vi "Autonomous Independent.vi"() -> ()   [LabVIEW 2014]
doc: "This VI is called when autonomous begins, and will automatically be terminated when autonomous ends. You can carry out timed or sensor driven robot movement independently without needing to return to the caller."
uses:
  Robot Global Data.vi
  <vilib>/Rock Robotics/Network Tables/NT Read Numeric Array.vi
  900/SwerveDrive/SwerveDriveRotate.vi
  <vilib>/Rock Robotics/WPI/CAN/TalonSRX/WPI_CANTalonSRX_APIControlMode.ctl
  <vilib>/Rock Robotics/Network Tables/NT Read Boolean Array.vi
  <vilib>/Rock Robotics/Network Tables/NT Read Number.vi
  <vilib>/Rock Robotics/Network Tables/NT Read Boolean.vi
panel:
  in  "Reverse Pivot Limit":dbl=-512.0
  in  "Forward Pivot Limit":dbl
  in  "Target X":dbl=103.5 format="%#_13g"
  # "Be sure to right-click and choose Data Operations>>Make Current Value default if you want to save the array values with the VI"
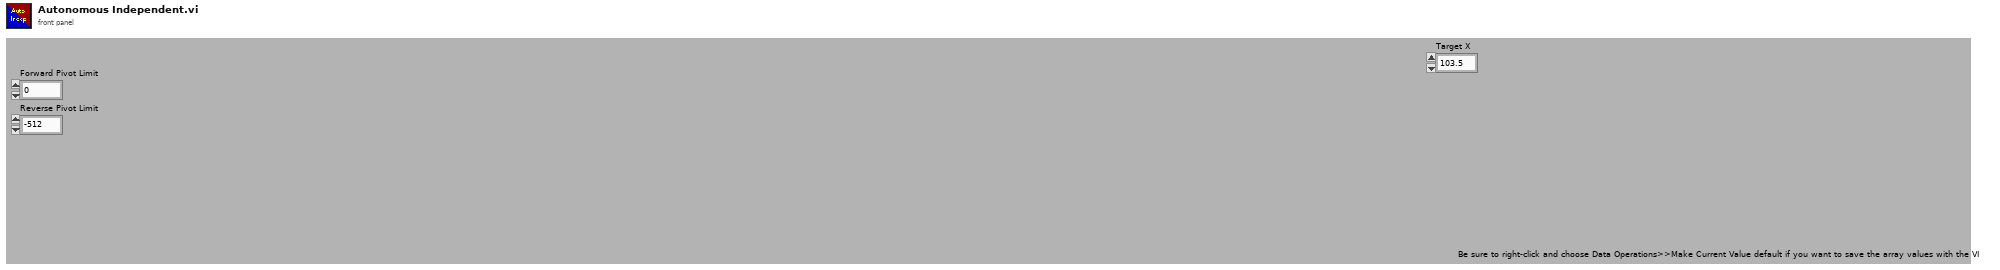
[diagram p1: front panel]
types:
  T1 = enum16{"Open", "Close", "Continue", "Stop", "Toggle"}
  T2 = typedef "WPI_CANTalonSRX_APIControlMode.ctl" = enum8{"Percent VBus", "Speed", "Position", "Slave", "Unchanged / Invalid"}
  T3 = typedef "WPI_MotorControlDeviceRef.ctl" = cluster{"DeviceStatus":errorcluster, "Type":T4, "PWM":cluster{"Controller":T5, "PWM Channel":T6, "DeadBand":T7}, "CAN":cluster{"Device Number":u8, "Control Mode":T8, "Semaphore":T9, "Max Vout":dbl, "TalonSRX Control Mode":T2}, "Invert":bool, "TransformRef":T10, "InvTransformRef":T10}
  T4 = typedef "WPI_MotorControlType.ctl" = enum16{"PWM", "CAN", "CANTalonSRX"}
  T5 = typedef "FPGA_TypedefDigitalModule.ctl" = enum16{"Controller 1"}
  T6 = typedef "FPGA_DIOPWMChannel.ctl" = enum8{"PWM 0", "PWM 1", "PWM 2", "PWM 3", "PWM 4", "PWM 5", "PWM 6", "PWM 7", "PWM 8", "PWM 9", "PWM MXP 0", "PWM MXP 1", "PWM MXP 2", "PWM MXP 3", "PWM MXP 4", "PWM MXP 5", "PWM MXP 6", "PWM MXP 7", "PWM MXP 8", "PWM MXP 9", "Invalid"}
  T7 = typedef "WPI_PWMDeadband.ctl" = cluster{"Name":string, "maxPositivePwm":i32, "minPositivePwm":i32, "centerPwm":i32, "maxNegativePwm":i32, "minNegativePwm":i32, "angularRange":u16}
  T8 = typedef "WPI_CANJaguar_ControlMode.ctl" = enum8{"Percent VBus", "Current", "Speed", "Position", "Voltage"}
  T9 = typedef "Semaphore RefNum" = refnum<k1>
  T10 = typedef "WPI_PWMTransform_ConPane.ctl" = refnum<vi>
  T11 = typedef "WPI_CANTalonSRX_GlobalStatus.ctl" = cluster{"Applied Throttle":dbl, "Module Enabled":bool, "CAN Error":errorcluster, "Closed Loop Error":dbl, "Forward Limit Switch Closed":bool, "Reverse Limit Switch Closed":bool, "Sensor Position":dbl, "Sensor Velocity":dbl, "Current":dbl, "Sticky Fault - Over Temp":bool, "Sticky Fault - Under Voltage":bool, "Sticky Fault - Forward Limit":bool, "Sticky Fault - Reverse Limit":bool, "Sticky Fault - Forward Soft Limit":bool, "Sticky Fault - Reverse Soft Limit":bool, "Brake is Enabled":bool, "Encoder Position":dbl, "Encoder Velocity":dbl, "Encoder Index Count":dbl, "Encoder A Pin State":bool, "Encoder B Pin State":bool, "Encoder Index Pin State":bool, "Analog In":dbl, "Analog In Velocity":dbl, "Temperature (C)":dbl, "Battery Voltage":dbl}
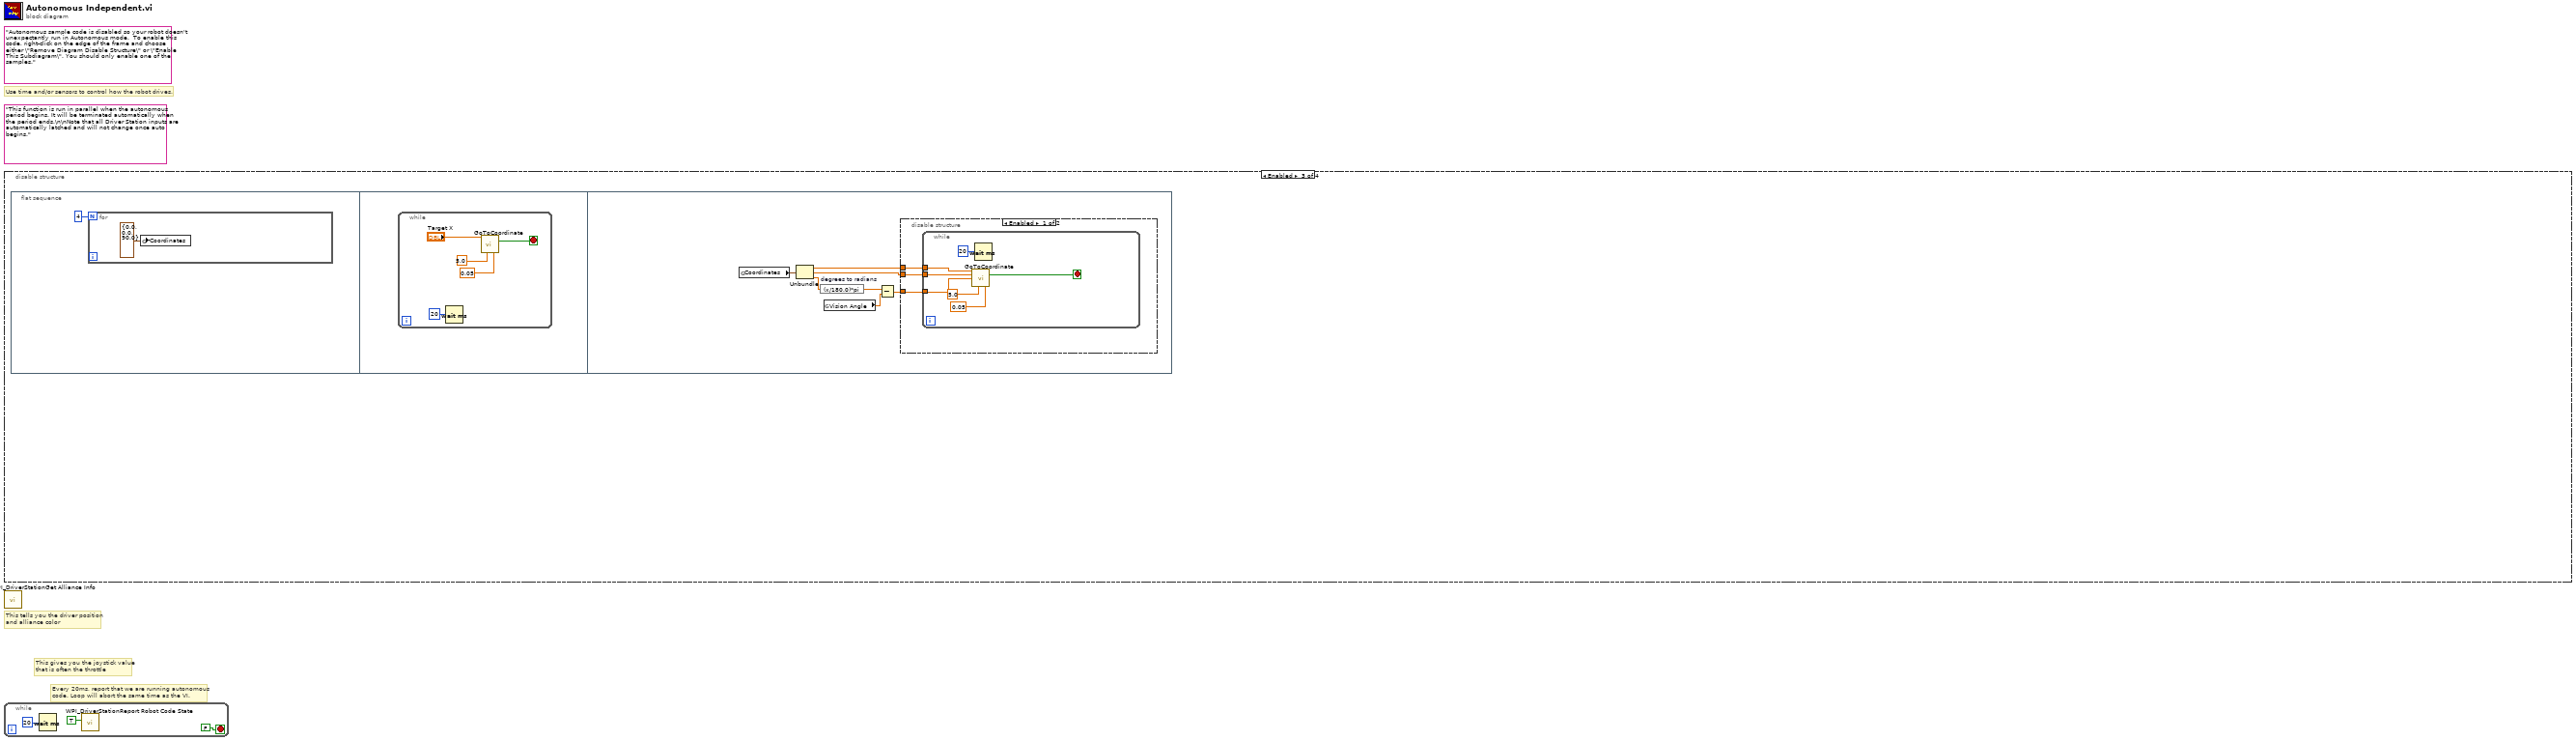
[diagram p0: block diagram]
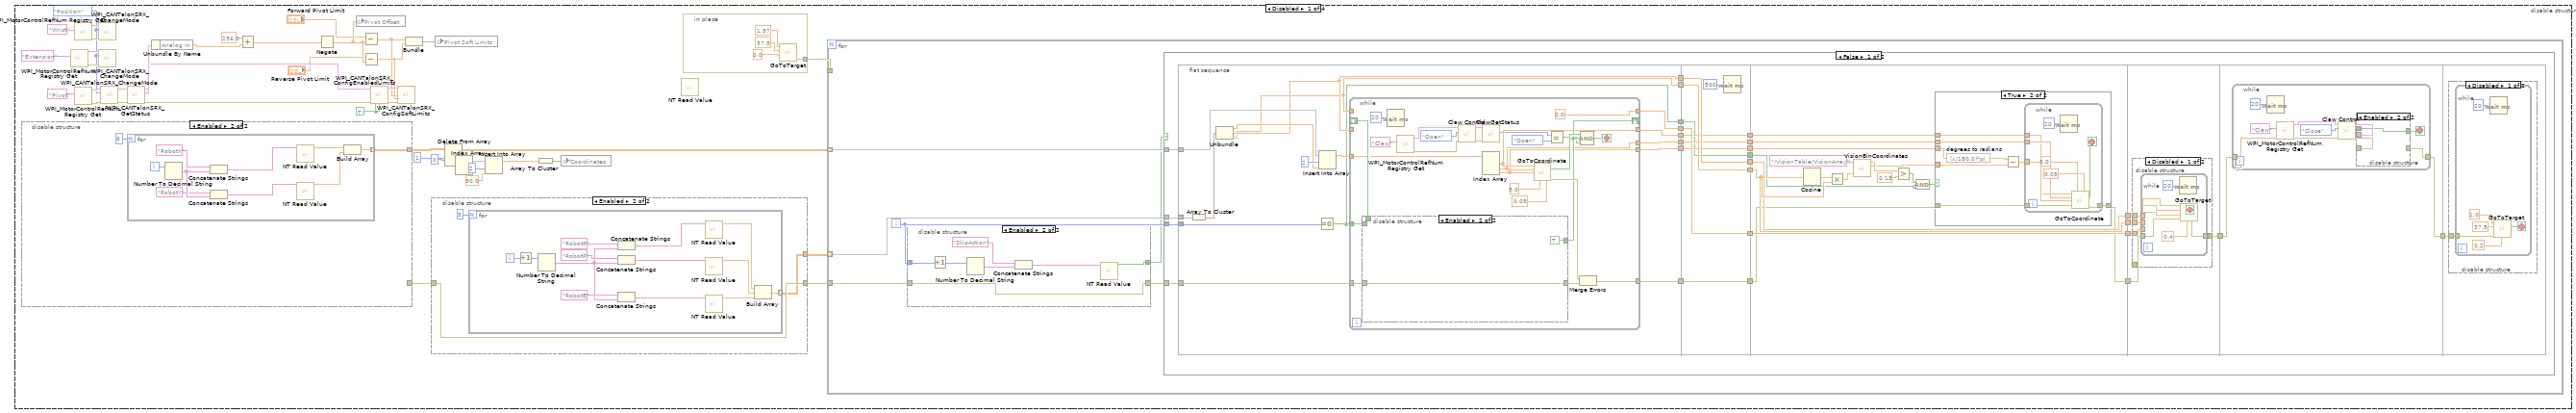
[diagram p2: hidden frame]
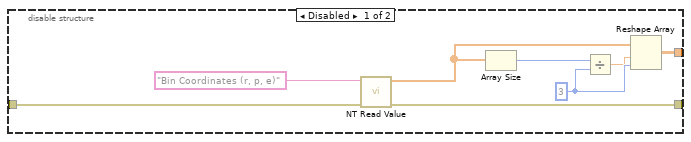
[diagram p3: hidden frame]
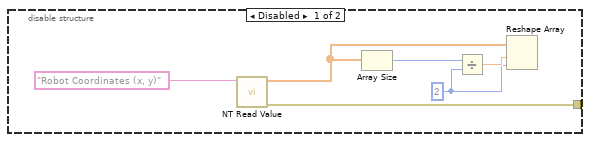
[diagram p4: hidden frame]
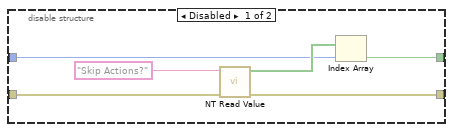
[diagram p5: hidden frame]
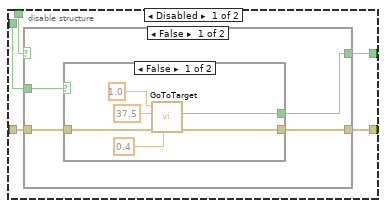
[diagram p6: hidden frame]
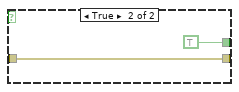
[diagram p7: hidden frame]
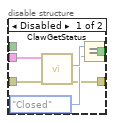
[diagram p11: hidden frame]
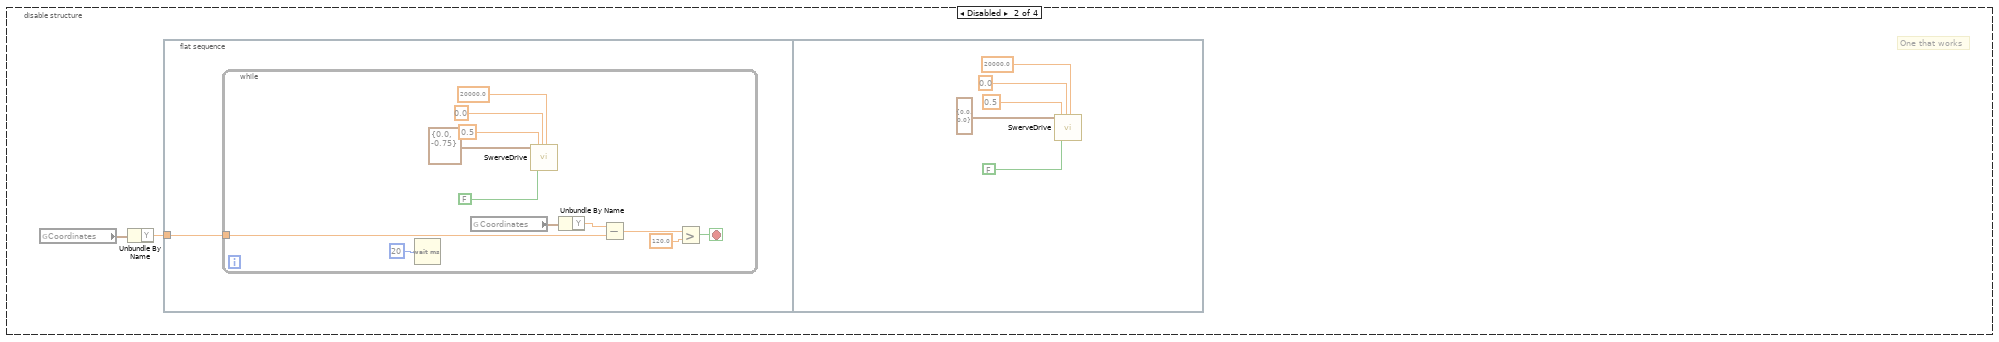
[diagram p14: hidden frame]
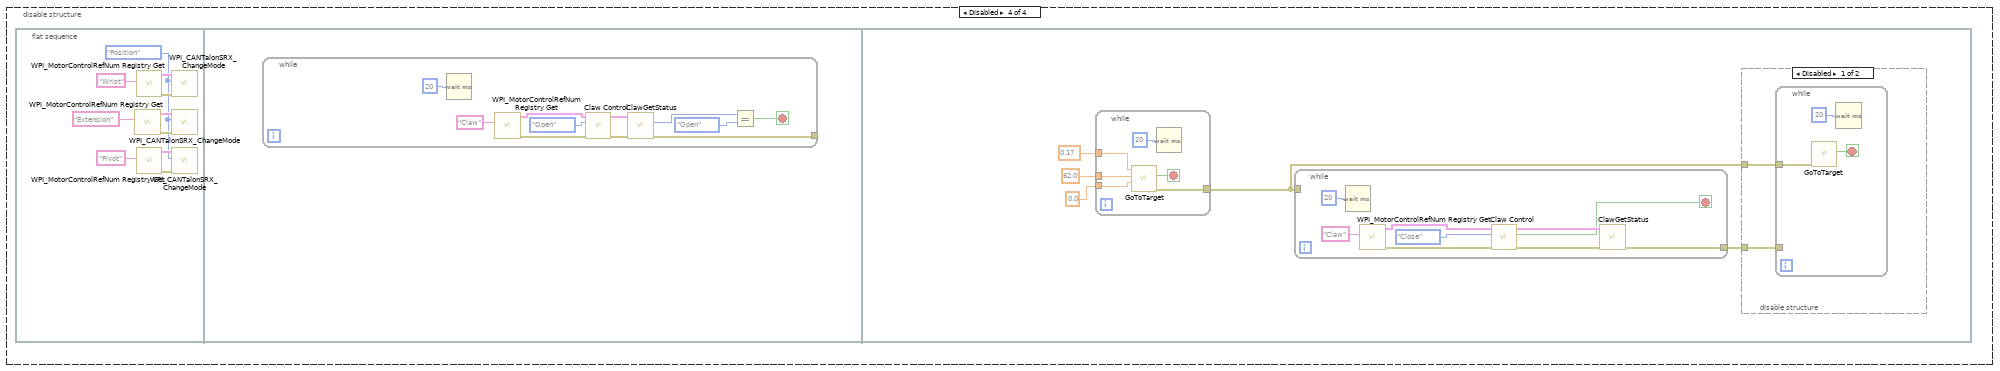
[diagram p16: hidden frame]
diagram:
  (unwired) "Autonomous sample code is disabled so your robot doesn't unexpectantly run in Autonomous mode.  To enable this code, right-click on the edge of the frame and choose either \"Remove Diagram Disable Structure\" or \"Enable This Subdiagram\". You should only enable one of the samples."
  (unwired) "This function is run in parallel when the autonomous period begins. It will be terminated automatically when the period ends.\n\nNote that all Driver Station inputs are automatically latched and will not change once auto begins."
  # "Every 20ms, report that we are running autonomous\ncode. Loop will abort the same time as the VI."
  # "This gives you the joystick value\nthat is often the throttle"
  # "Use time and/or sensors to control how the robot drives."
  # "This tells you the driver position\nand alliance color"
  n1 = disable-structure shown="Enabled" {
    frame Disabled {
      w7 = TRUE ("Forward Soft Limit Enable")
      w22 = WPI_CANTalonSRX_APIControlMode."Position" ("Control Mode")
      n2 = disable-structure shown="Enabled" {
        disable-tunnel: [_ w77] -> w20
        disable-tunnel: [w74 _] -> w37
        frame Disabled {
          w72 = 2 ("dimension size")
          n3 = call-poly <vilib>:"NT Read Value.vi"("Name"="Robot Coordinates (x, y)") -> ("error out"=w74:errorcluster, "Numeric Array"=w70:dbl[])  [unwired: 9 in]
          n4 = Array Size(array=w70) -> (size(s)=w71:i32)
          n5 = Divide(x=w71, y=w72) -> (x/y=w73:dbl)
          n6 = Reshape Array(w70, w73, w72) -> ()  [unwired: 1 out]
        }
        frame Enabled {
          n7 = for {
            N: 6 -> [_]
            tunnel: [w78] -> w77 mode=indexing
            i -> [w84]
            n8 = Number To Decimal String(number=w84) -> (decimal integer string=w82:string)  [unwired: 1 in]
            n9 = Concatenate Strings("RobotX" ("string"), w82) -> (w86:string)
            n10 = Concatenate Strings("RobotY" ("string"), w82) -> (w83:string)
            n11 = call-poly <vilib>:"NT Read Value.vi"("Name"=w86) -> ("Numeric"=w80:dbl)  [unwired: 9 in, 1 out]
            n12 = call-poly <vilib>:"NT Read Value.vi"("Name"=w83) -> ("Numeric"=w79:dbl)  [unwired: 9 in, 1 out]
            n13 = Build Array(w80, w79) -> (w78:dbl[])
          }
        }
      }
      n14 = call <vilib>:"WPI_MotorControlRefNum Registry Get.vi"("refnum name"="Extension") -> ("error out"=w24:errorcluster, "MotorControlDevRef"=w23:T3)  [unwired: 9 in]
      n15 = call <vilib>:"WPI_MotorControlRefNum Registry Get.vi"("refnum name"="Wrist") -> ("error out"=w27:errorcluster, "MotorControlDevRef"=w26:T3)  [unwired: 9 in]
      n16 = call <vilib>:"WPI_MotorControlRefNum Registry Get.vi"("refnum name"="Pivot") -> ("error out"=w30:errorcluster, "MotorControlDevRef"=w29:T3)  [unwired: 9 in]
      n17 = call <vilib>:"WPI_CANTalonSRX_ChangeMode.vi"("error in (no error)"=w27, "Control Mode"=w22, "CAN Talon SRX Ref"=w26) -> ()  [unwired: 7 in, 2 out]
      n18 = call <vilib>:"WPI_CANTalonSRX_ChangeMode.vi"("error in (no error)"=w24, "Control Mode"=w22, "CAN Talon SRX Ref"=w23) -> ()  [unwired: 7 in, 2 out]
      n19 = call <vilib>:"WPI_CANTalonSRX_ChangeMode.vi"("error in (no error)"=w30, "Control Mode"=w22, "CAN Talon SRX Ref"=w29) -> ("error out"=w11:errorcluster, "CAN Talon SRX Ref Out"=w10:T3)  [unwired: 7 in]
      n20 = call <vilib>:"WPI_CANTalonSRX_GetStatus.vi"("error in (no error)"=w11, "CAN Talon SRX Ref"=w10) -> ("error out"=w14:errorcluster, "Talon SRX Status"=w13:T11, "CAN Talon SRX Ref Out"=w12:T3)  [unwired: 7 in]
      n21 = Unbundle By Name(w13) -> ("Analog In"=w15:dbl)
      n22 = Add(x=256.0, y=w15) -> (x+y=w16:dbl)
      n23 = Negate(x=w16) -> (-x=w17:dbl)
      n24 = global write "Robot Global Data.vi" "Pivot Offset"(w17) -> ()
      n25 = Subtract(x="Forward Pivot Limit", y=w17) -> (x-y=w6:dbl)
      n26 = Subtract(x="Reverse Pivot Limit", y=w17) -> (x-y=w18:dbl)
      n27 = call <vilib>:"WPI_CANTalonSRX_ConfigEnabledLimits.vi"("CAN Talon SRX Ref"=w12, "error in (no error)"=w14, "Forward Soft Limit Enable"=w7, "Reverse Soft Limit Enable"=w7) -> ("CAN Talon SRX Ref Out"=w9:T3, "error out"=w8:errorcluster)  [unwired: 10 in]
      n28 = call <vilib>:"WPI_CANTalonSRX_ConfigSoftLimits.vi"("CAN Talon SRX Ref"=w9, "Forward Limit Position"=w6, "Reverse Limit Position"=w18, "error in (no error)"=w8) -> ()  [unwired: 10 in, 2 out]
      n29 = Bundle(w6, w18) -> (w19:cluster{dbl, dbl})  [unwired: 1 in]
      n30 = disable-structure shown="Enabled" {
        disable-tunnel: [w44 w50] -> w39
        disable-tunnel: [w43 w51] -> w38
        disable-tunnel: w37 -> [w42 w51]
        frame Disabled {
          w46 = 3 ("dimension size")
          n31 = call-poly <vilib>:"NT Read Value.vi"("error in"=w42, "Name"="Bin Coordinates (r, p, e)") -> ("error out"=w43:errorcluster, "Numeric Array"=w48:dbl[])  [unwired: 8 in]
          n32 = Array Size(array=w48) -> (size(s)=w47:i32)
          n33 = Divide(x=w47, y=w46) -> (x/y=w45:dbl)
          n34 = Reshape Array(w48, w45, w46) -> (w44:dbl[][])
        }
        frame Enabled {
          n35 = for {
            N: 5 -> [_]
            tunnel: [w58] -> w50 mode=indexing
            i -> [w63]
            n36 = Increment(x=w63) -> (x+1=w53:i32)
            n37 = Number To Decimal String(number=w53) -> (decimal integer string=w54:string)  [unwired: 1 in]
            n38 = Concatenate Strings("RobotR" ("string"), w54) -> (w65:string)
            n39 = Concatenate Strings("RobotP" ("string"), w54) -> (w62:string)
            n40 = Concatenate Strings("RobotE" ("string"), w54) -> (w57:string)
            n41 = call-poly <vilib>:"NT Read Value.vi"("Name"=w65) -> ("Numeric"=w60:dbl)  [unwired: 9 in, 1 out]
            n42 = call-poly <vilib>:"NT Read Value.vi"("Name"=w62) -> ("Numeric"=w59:dbl)  [unwired: 9 in, 1 out]
            n43 = call-poly <vilib>:"NT Read Value.vi"("Name"=w57) -> ("Numeric"=w55:dbl)  [unwired: 9 in, 1 out]
            n44 = Build Array(w60, w59, w55) -> (w58:dbl[])
          }
        }
      }
      n45 = global write "Robot Global Data.vi" "Pivot Soft Limits"(w19) -> ()
      n46 = Delete From Array(array=w20, length=1, index (row)=0) -> (deleted portion=w34:dbl[][], array with subset deleted=w40:dbl[][])  [unwired: 1 in]
      n47 = Index Array(array=w34) -> (element=w1:dbl[])  [unwired: 2 in]
      n48 = Insert Into Array(array=w1, index=2, new element=90.0 ("new element/subarray")) -> (w35:dbl[])
      n49 = Array To Cluster(array=w35) -> (cluster=w36:cluster{"[0]":dbl, "[1]":dbl, "[2]":dbl})
      n50 = global write "Robot Global Data.vi" "Coordinates"(w36) -> ()
      n51 = call-poly <vilib>:"NT Read Value.vi"() -> ()  [unwired: 10 in, 2 out]
      n52 = in-place {
        in-place-border: [w67] -> w21
        n53 = call "GoToTarget.vi"("target wrist angle (rad; relative to ground)"=0.0, "target extension (in.)"=37.5, "target arm angle (rad)"=1.57) -> ("error out"=w67:errorcluster)  [unwired: 7 in, 1 out]
      }
      n54 = for {
        tunnel: w40 -> [w92] mode=indexing
        tunnel: w39 -> [w91] mode=indexing
        tunnel: w38 -> [w89]
        tunnel: w21 -> [_]
        i -> [w88]
        n55 = disable-structure shown="Enabled" {
          disable-tunnel: [w97 w99] -> w90
          disable-tunnel: w89 -> [w96 w99]
          disable-tunnel: w88 -> [w93 w102]
          disable-tunnel: [w94 w100] -> w87
          frame Disabled {
            n56 = call-poly <vilib>:"NT Read Value.vi"("error in"=w96, "Name"="Skip Actions?") -> ("error out"=w97:errorcluster, "Boolean Array"=w95:bool[])  [unwired: 8 in]
            n57 = Index Array(array=w95, index=w93) -> (element=w94:bool)
          }
          frame Enabled {
            n58 = Increment(x=w102) -> (x+1=w103:i32)
            n59 = Number To Decimal String(number=w103) -> (decimal integer string=w104:string)  [unwired: 1 in]
            n60 = Concatenate Strings("SkipAction" ("string"), w104) -> (w105:string)
            n61 = call-poly <vilib>:"NT Read Value.vi"("Name"=w105) -> ("Boolean"=w100:bool)  [unwired: 9 in, 1 out]
          }
        }
        n62 = case shown="False" w87 {
          tunnel: w92 -> [w131 _]
          tunnel: w91 -> [w130 _]
          tunnel: w90 -> [w129 _]
          tunnel: w88 -> [w128 _]
          frame False {
            n63 = flat-sequence {
              tunnel: w131 -> [w145]
              tunnel: w130 -> [w147]
              tunnel: [w138] -> w121
              tunnel: [w142] -> w119
              tunnel: [w141] -> w117
              tunnel: [w140] -> w115
              tunnel: w128 -> [w133]
              tunnel: w129 -> [w139]
              tunnel: [w136] -> w113
              tunnel: [w135] -> w111
              tunnel: [w134] -> w109
              tunnel: [w132] -> w107
              tunnel: w121 -> [w203]
              tunnel: [w203] -> w120
              tunnel: w119 -> [w202]
              tunnel: [w202] -> w118
              tunnel: w117 -> [w201]
              tunnel: [w201] -> w116
              tunnel: w115 -> [w200]
              tunnel: [w200] -> w114
              tunnel: w113 -> [w199]
              tunnel: [w199] -> w112
              tunnel: w111 -> [w198]
              tunnel: [w198] -> w110
              tunnel: w109 -> [w197]
              tunnel: [w197] -> w108
              tunnel: w107 -> [w196]
              tunnel: [w196] -> w106
              tunnel: w120 -> [w220]
              tunnel: [w220] -> w125
              tunnel: w118 -> [w204]
              tunnel: [w205] -> w124
              tunnel: w116 -> [w219]
              tunnel: [w219] -> w123
              tunnel: w114 -> [w218]
              tunnel: [w218] -> w122
              tunnel: w112 -> [w217]
              tunnel: w110 -> [w216]
              tunnel: w108 -> [w215]
              tunnel: w106 -> [w211]
              tunnel: w125 -> [w240]
              tunnel: w124 -> [w243]
              tunnel: w123 -> [w239]
              tunnel: w122 -> [w242]
              tunnel: [w241] -> w126
              tunnel: [w258] -> w127
              tunnel: w126 -> [w259]
              tunnel: w127 -> [w278]
              frame #0 {
                n64 = Array To Cluster(array=w147) -> (cluster=w146:cluster{"[0]":dbl, "[1]":dbl, "[2]":dbl})
                n65 = Unbundle(w146) -> ("[0]"=w143:dbl, "[1]"=w141:dbl, "[2]"=w138:dbl)
                n66 = Insert Into Array(array=w145, index=2, new element=w143) -> (w137:dbl[])
                n67 = Equal To 0?(x=w133) -> (x = 0?=w132:bool)
                n68 = while {
                  tunnel: [w173] -> w142
                  tunnel: w141 -> [_]
                  tunnel: [0.0 ("target wrist angle (rad; relative to ground)")] -> w140
                  shift-right: [w168] -> _
                  shift-left: _ -> [w165]
                  tunnel: w139 -> [w170]
                  tunnel: w138 -> [_]
                  tunnel: w137 -> [w164]
                  tunnel: [w163] -> w136
                  tunnel: [w162] -> w135
                  tunnel: [w161] -> w134
                  tunnel: w132 -> [w157]
                  stop <- w167 stop-if-true
                  n69 = disable-structure shown="Enabled" {
                    disable-tunnel: w170 -> [w178 w193]
                    disable-tunnel: [w177 TRUE ("finished")] -> w168
                    disable-tunnel: w165 -> [w176 _]
                    disable-tunnel: [w175 w193] -> w159
                    disable-tunnel: w157 -> [w174 _]
                    frame Disabled {
                      n70 = case shown="False" w176 {
                        selector: w176 -> [_ w192]
                        tunnel: [w182 w192] -> w177
                        tunnel: [w181 w191] -> w175
                        tunnel: w178 -> [w180 w191]
                        tunnel: w174 -> [w179 _]
                        frame False {
                          n71 = case shown="False" w179 {
                            tunnel: [w188 TRUE] -> w182
                            tunnel: [w187 w189] -> w181
                            tunnel: w180 -> [w186 w189]
                            frame False {
                              n72 = call "GoToTarget.vi"("Extension Power"=0.4, "error in (no error)"=w186, "target extension (in.)"=37.5, "target arm angle (rad)"=1.0) -> ("error out"=w187:errorcluster, "finished"=w188:bool)  [unwired: 6 in]
                            }
                            frame True {
                            }
                          }
                        }
                        frame True {
                        }
                      }
                    }
                    frame Enabled {
                    }
                  }
                  n73 = Wait (ms)(milliseconds to wait=u32 20) -> ()  [unwired: 1 out]
                  n74 = call <vilib>:"WPI_MotorControlRefNum Registry Get.vi"("refnum name"="Claw") -> ("error out"=w155:errorcluster, "MotorControlDevRef"=w154:T3)  [unwired: 9 in]
                  n75 = call "Claw Control.vi"("error in (no error)"=w155, "Operation"=T1."Open", "MotorControlDevRef"=w154) -> ("error out"=w151:errorcluster, "MotorControlDevRef"=w150:T3)  [unwired: 4 in, 1 out]
                  n76 = call "ClawGetStatus.vi"("error in (no error)"=w151, "MotorControlDevRef"=w150) -> ("Claw State"=w149:enum16{"Open", "Closed", "Neither"})  [unwired: 5 in, 4 out]
                  n77 = Index Array(array=w164) -> (element #1=w163:dbl, element #2=w162:dbl, element #3=w161:dbl)  [unwired: 3 in]
                  n78 = call "GoToCoordinate.vi"("Target X"=w163, "Target Y"=w162, "Target Angle (rad)"=w161, "Position Tolerance"=5.0, "Angle Tolerance"=0.05) -> ("Finished"=w169:bool, "error out"=w172:errorcluster)  [unwired: 9 in]
                  n79 = Equal?(x=w149, y=enum16{"Open", "Closed", "Neither"}."Open") -> (x = y?=w158:bool)
                  n80 = Merge Errors(w172, w159) -> (w173:errorcluster)
                  n81 = Compound Arithmetic op=AND(w169, w168, w158) -> (w167:bool)
                }
              }
              frame #1 {
                n82 = Wait (ms)(milliseconds to wait=u32 500) -> ()  [unwired: 1 out]
              }
              frame #2 {
                n83 = Cosine(x=w220) -> (cos(x)=w206:dbl)
                n84 = Multiply(x=w206, y=w220) -> (x*y=w207:dbl)
                n85 = call "VisionBinCoordinates.vi"("Vision Array Name"="/VisionTable/VisionArray", "Distance to Bin"=w207) -> ("bin ratio"=w209:dbl, "bin angle"=w208:dbl)  [unwired: 1 in, 2 out]
                n86 = Greater?(x=w209, y=0.15) -> (0:w214:bool)
                n87 = Compound Arithmetic op=AND(w214, invert w211) -> (w212:bool)
                n88 = case shown="True" w212 {
                  tunnel: w217 -> [_ w227]
                  tunnel: w216 -> [_ w226]
                  tunnel: w215 -> [_ w225]
                  tunnel: w208 -> [_ w224]
                  tunnel: [w221 w222] -> w205
                  tunnel: w204 -> [w221 w223]
                  frame False {
                  }
                  frame True {
                    n89 = expression code="(x/180.0)*pi" "degrees to radians"(w225) -> (w229:dbl)
                    n90 = Subtract(x=w229, y=w224) -> (x-y=w228:dbl)
                    n91 = while {
                      tunnel: w228 -> [w234]
                      tunnel: w226 -> [w233]
                      tunnel: w227 -> [w232]
                      tunnel: w223 -> [w230]
                      tunnel: [w231] -> w222
                      stop <- w235 stop-if-true
                      n92 = Wait (ms)(milliseconds to wait=u32 20) -> ()  [unwired: 1 out]
                      n93 = call "GoToCoordinate.vi"("Target X"=w232, "Target Y"=w233, "Target Angle (rad)"=w234, "error in (no error)"=w230, "Position Tolerance"=5.0, "Angle Tolerance"=0.05) -> ("Finished"=w235:bool, "error out"=w231:errorcluster)  [unwired: 8 in]
                    }
                  }
                }
              }
              frame #3 {
                n94 = disable-structure shown="Disabled" {
                  disable-tunnel: w243 -> [w248 w257]
                  disable-tunnel: w242 -> [w247 _]
                  disable-tunnel: [w246 w257] -> w241
                  disable-tunnel: w240 -> [w245 _]
                  disable-tunnel: w239 -> [w244 _]
                  frame Disabled {
                    n95 = while {
                      tunnel: w245 -> [w256]
                      tunnel: w248 -> [w255]
                      tunnel: w244 -> [w254]
                      tunnel: w247 -> [w253]
                      tunnel: [w250] -> w246
                      stop <- w252 stop-if-true
                      n96 = Wait (ms)(milliseconds to wait=u32 20) -> ()  [unwired: 1 out]
                      n97 = call "GoToTarget.vi"("Extension Power"=0.4, "error in (no error)"=w255, "target wrist angle (rad; relative to ground)"=w253, "target extension (in.)"=w256, "target arm angle (rad)"=w254) -> ("error out"=w250:errorcluster, "finished"=w252:bool)  [unwired: 5 in]
                    }
                  }
                  frame Enabled {
                  }
                }
              }
              frame #4 {
                n98 = while {
                  tunnel: w259 -> [w262]
                  tunnel: [w261] -> w258
                  stop <- w263 stop-if-true
                  n99 = Wait (ms)(milliseconds to wait=u32 20) -> ()  [unwired: 1 out]
                  n100 = call <vilib>:"WPI_MotorControlRefNum Registry Get.vi"("error in (no error)"=w262, "refnum name"="Claw") -> ("error out"=w269:errorcluster, "MotorControlDevRef"=w266:T3)  [unwired: 8 in]
                  n101 = call "Claw Control.vi"("error in (no error)"=w269, "Operation"=T1."Close", "MotorControlDevRef"=w266) -> ("error out"=w265:errorcluster, "Holding"=w260:bool, "MotorControlDevRef"=w264:T3)  [unwired: 4 in]
                  n102 = disable-structure shown="Enabled" {
                    disable-tunnel: w265 -> [w276 _]
                    disable-tunnel: w264 -> [w275 _]
                    disable-tunnel: [w272 w277] -> w263
                    disable-tunnel: [w271 _] -> w261
                    disable-tunnel: w260 -> [_ w277]
                    frame Disabled {
                      n103 = call "ClawGetStatus.vi"("error in (no error)"=w276, "MotorControlDevRef"=w275) -> ("error out"=w271:errorcluster, "Claw State"=w274:enum16{"Open", "Closed", "Neither"})  [unwired: 5 in, 3 out]
                      n104 = Equal?(x=w274, y=enum16{"Open", "Closed", "Neither"}."Closed") -> (x = y?=w272:bool)
                    }
                    frame Enabled {
                    }
                  }
                }
              }
              frame #5 {
                n105 = disable-structure shown="Disabled" {
                  disable-tunnel: w278 -> [w279 _]
                  frame Disabled {
                    n106 = while {
                      tunnel: w279 -> [w285]
                      stop <- w284 stop-if-true
                      n107 = Wait (ms)(milliseconds to wait=u32 20) -> ()  [unwired: 1 out]
                      n108 = call "GoToTarget.vi"("Extension Power"=0.2, "error in (no error)"=w285, "target extension (in.)"=37.5, "target arm angle (rad)"=1.0) -> ("finished"=w284:bool)  [unwired: 6 in, 1 out]
                    }
                  }
                  frame Enabled {
                  }
                }
              }
            }
          }
          frame True {
          }
        }
      }
    }
    frame Disabled {
      # "One that works"
      n109 = global read "Robot Global Data.vi" "Coordinates"() -> (w287:cluster{"X":dbl, "Y":dbl, "Heading":dbl})
      n110 = Unbundle By Name(w287) -> ("Y"=w286:dbl)
      n111 = flat-sequence {
        tunnel: w286 -> [w288]
        frame #0 {
          n112 = while {
            tunnel: w288 -> [w294]
            stop <- w293 stop-if-true
            n113 = Wait (ms)(milliseconds to wait=u32 20) -> ()  [unwired: 1 out]
            n114 = global read "Robot Global Data.vi" "Coordinates"() -> (w296:cluster{"X":dbl, "Y":dbl, "Heading":dbl})
            n115 = call-poly "SwerveDrive.vi"("Strafe Joystick Axes"=cluster{"Left":dbl, "Right":dbl} {"Left"=0.0, "Right"=-0.75} ("Trigger Axes"), "Strafe Multiplier"=0.5, "FieldCentric? (T)"=FALSE, "Rotation Multiplier"=0.0, "Max Wheel Speed"=20000.0) -> ()  [unwired: 12 in, 3 out]
            n116 = Unbundle By Name(w296) -> ("Y"=w295:dbl)
            n117 = Subtract(x=w295, y=w294) -> (x-y=w292:dbl)
            n118 = Greater?(x=w292, y=120.0 ("x")) -> (0:w293:bool)
          }
        }
        frame #1 {
          n119 = call-poly "SwerveDrive.vi"("Strafe Joystick Axes"=cluster{"Left":dbl, "Right":dbl} {"Left"=0.0, "Right"=0.0} ("Trigger Axes"), "Strafe Multiplier"=0.5, "FieldCentric? (T)"=FALSE, "Rotation Multiplier"=0.0, "Max Wheel Speed"=20000.0) -> ()  [unwired: 12 in, 3 out]
        }
      }
    }
    frame Enabled {
      n120 = flat-sequence {
        frame #0 {
          n121 = for {
            N: 4 -> [_]
            n122 = global write "Robot Global Data.vi" "Coordinates"(cluster{"X":dbl, "Y":dbl, "Heading":dbl} {"X"=0.0, "Y"=0.0, "Heading"=90.0} ("Coordinates")) -> ()
          }
        }
        frame #1 {
          n123 = while {
            stop <- w308 stop-if-true
            n124 = Wait (ms)(milliseconds to wait=u32 20) -> ()  [unwired: 1 out]
            n125 = call "GoToCoordinate.vi"("Target X"="Target X", "Position Tolerance"=5.0, "Angle Tolerance"=0.05) -> ("Finished"=w308:bool)  [unwired: 11 in, 1 out]
          }
        }
        frame #2 {
          n126 = global read "Robot Global Data.vi" "Coordinates"() -> (w316:cluster{"X":dbl, "Y":dbl, "Heading":dbl})
          n127 = Unbundle(w316) -> ("X"=w313:dbl, "Y"=w314:dbl, "Heading"=w317:dbl)
          n128 = expression code="(x/180.0)*pi" "degrees to radians"(w317) -> (w318:dbl)
          n129 = global read "Robot Global Data.vi" "Vision Angle"() -> (w319:dbl)
          n130 = Subtract(x=w318, y=w319) -> (x-y=w315:dbl)
          n131 = disable-structure shown="Enabled" {
            disable-tunnel: w315 -> [w322 _]
            disable-tunnel: w314 -> [w321 _]
            disable-tunnel: w313 -> [w320 _]
            frame Enabled {
              n132 = while {
                tunnel: w322 -> [w325]
                tunnel: w321 -> [w324]
                tunnel: w320 -> [w323]
                stop <- w326 stop-if-true
                n133 = call "GoToCoordinate.vi"("Target X"=w323, "Target Y"=w324, "Target Angle (rad)"=w325, "Position Tolerance"=5.0, "Angle Tolerance"=0.05) -> ("Finished"=w326:bool)  [unwired: 9 in, 1 out]
                n134 = Wait (ms)(milliseconds to wait=u32 20) -> ()  [unwired: 1 out]
              }
            }
            frame Disabled {
            }
          }
        }
      }
    }
    frame Disabled {
      n135 = flat-sequence {
        frame #0 {
          w330 = WPI_CANTalonSRX_APIControlMode."Position" ("Control Mode")
          n136 = call <vilib>:"WPI_MotorControlRefNum Registry Get.vi"("refnum name"="Extension") -> ("error out"=w332:errorcluster, "MotorControlDevRef"=w331:T3)  [unwired: 9 in]
          n137 = call <vilib>:"WPI_MotorControlRefNum Registry Get.vi"("refnum name"="Wrist") -> ("error out"=w335:errorcluster, "MotorControlDevRef"=w334:T3)  [unwired: 9 in]
          n138 = call <vilib>:"WPI_MotorControlRefNum Registry Get.vi"("refnum name"="Pivot") -> ("error out"=w338:errorcluster, "MotorControlDevRef"=w337:T3)  [unwired: 9 in]
          n139 = call <vilib>:"WPI_CANTalonSRX_ChangeMode.vi"("error in (no error)"=w335, "Control Mode"=w330, "CAN Talon SRX Ref"=w334) -> ()  [unwired: 7 in, 2 out]
          n140 = call <vilib>:"WPI_CANTalonSRX_ChangeMode.vi"("error in (no error)"=w332, "Control Mode"=w330, "CAN Talon SRX Ref"=w331) -> ()  [unwired: 7 in, 2 out]
          n141 = call <vilib>:"WPI_CANTalonSRX_ChangeMode.vi"("error in (no error)"=w338, "Control Mode"=w330, "CAN Talon SRX Ref"=w337) -> ()  [unwired: 7 in, 2 out]
        }
        frame #1 {
          n142 = while {
            tunnel: [w340] -> _
            stop <- w341 stop-if-true
            n143 = Wait (ms)(milliseconds to wait=u32 20) -> ()  [unwired: 1 out]
            n144 = call <vilib>:"WPI_MotorControlRefNum Registry Get.vi"("refnum name"="Claw") -> ("error out"=w349:errorcluster, "MotorControlDevRef"=w346:T3)  [unwired: 9 in]
            n145 = call "Claw Control.vi"("error in (no error)"=w349, "Operation"=T1."Open", "MotorControlDevRef"=w346) -> ("error out"=w345:errorcluster, "MotorControlDevRef"=w344:T3)  [unwired: 4 in, 1 out]
            n146 = call "ClawGetStatus.vi"("error in (no error)"=w345, "MotorControlDevRef"=w344) -> ("error out"=w340:errorcluster, "Claw State"=w343:enum16{"Open", "Closed", "Neither"})  [unwired: 5 in, 3 out]
            n147 = Equal?(x=w343, y=enum16{"Open", "Closed", "Neither"}."Open") -> (x = y?=w341:bool)
          }
        }
        frame #2 {
          n148 = while {
            tunnel: 62.0 ("Numeric Array[2]") -> [w366]
            tunnel: 0.17 ("Numeric Array[1]") -> [w365]
            tunnel: 0.0 ("target wrist angle (rad; relative to ground)") -> [w364]
            tunnel: [w361] -> w355
            stop <- w363 stop-if-true
            n149 = call "GoToTarget.vi"("target wrist angle (rad; relative to ground)"=w364, "target extension (in.)"=w366, "target arm angle (rad)"=w365) -> ("error out"=w361:errorcluster, "finished"=w363:bool)  [unwired: 7 in]
            n150 = Wait (ms)(milliseconds to wait=u32 20) -> ()  [unwired: 1 out]
          }
          n151 = while {
            tunnel: w355 -> [_]
            tunnel: [w368] -> w354
            stop <- w367 stop-if-true
            n152 = Wait (ms)(milliseconds to wait=u32 20) -> ()  [unwired: 1 out]
            n153 = call <vilib>:"WPI_MotorControlRefNum Registry Get.vi"("refnum name"="Claw") -> ("error out"=w374:errorcluster, "MotorControlDevRef"=w371:T3)  [unwired: 9 in]
            n154 = call "Claw Control.vi"("error in (no error)"=w374, "Operation"=T1."Close", "MotorControlDevRef"=w371) -> ("error out"=w370:errorcluster, "Holding"=w367:bool, "MotorControlDevRef"=w369:T3)  [unwired: 4 in]
            n155 = call "ClawGetStatus.vi"("error in (no error)"=w370, "MotorControlDevRef"=w369) -> ("error out"=w368:errorcluster)  [unwired: 5 in, 4 out]
          }
          n156 = disable-structure shown="Disabled" {
            disable-tunnel: w355 -> [w357 _]
            disable-tunnel: w354 -> [w356 _]
            frame Disabled {
              n157 = while {
                tunnel: w357 -> [w360]
                tunnel: w356 -> [_]
                stop <- w359 stop-if-true
                n158 = call "GoToTarget.vi"("error in (no error)"=w360) -> ("finished"=w359:bool)  [unwired: 9 in, 1 out]
                n159 = Wait (ms)(milliseconds to wait=u32 20) -> ()  [unwired: 1 out]
              }
            }
            frame Enabled {
            }
          }
        }
      }
    }
  }
  n160 = call <vilib>:"WPI_DriverStationGet Alliance Info.vi"() -> ()  [unwired: 12 out]
  n161 = while {
    stop <- FALSE stop-if-true
    n162 = Wait (ms)(milliseconds to wait=u32 20) -> ()  [unwired: 1 out]
    n163 = call <vilib>:"WPI_DriverStationReport Robot Code State.vi"("Autonomous"=TRUE) -> ()  [unwired: 10 in, 1 out]
  }
